vi "get_ROI_boundary.vi"(8 "error in (no error)":errorcluster, 11 "image in":T2) -> (0 "error out":errorcluster, 2 "points":T1[](array[typedef]))   [LabVIEW 2010]
uses:
  <vilib>/vision/Image Controls.llb/IMAQ Image.ctl
  point_cluster.ctl
  <vilib>/vision/NI_Vision_Development_Module.lvlib
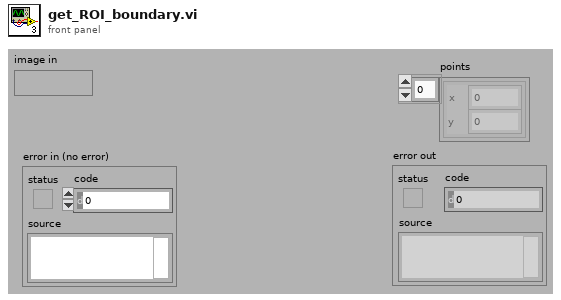
[diagram p1: front panel]
types:
  T1 = typedef "point_cluster.ctl" = cluster{"x":i32, "y":i32}
  T2 = typedef "IMAQ Image.ctl" = refnum<image>
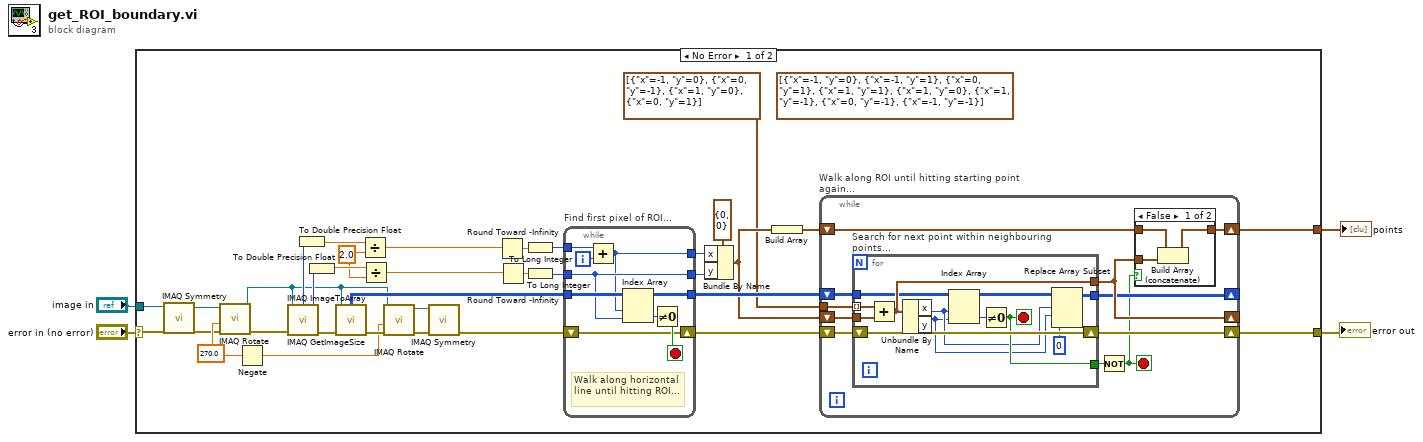
[diagram p0: block diagram]
diagram:
  n1 = case shown="No Error" "error in (no error)" {
    selector: "error in (no error)" -> [w15 w74]
    tunnel: [w26 w74] -> w3
    tunnel: "image in" -> [w13 _]
    tunnel: [w8 _] -> w1
    frame No Error {
      w17 = sgl 270.0 ("Angle (degrees)")
      (unwired) T1[] [{"x"=-1, "y"=0}, {"x"=-1, "y"=1}, {"x"=0, "y"=1}, {"x"=1, "y"=1}, {"x"=1, "y"=0}, {"x"=1, "y"=-1}, {"x"=0, "y"=-1}, {"x"=-1, "y"=-1}]
      w32 = 2.0 ("y")
      n2 = call "IMAQ Symmetry"("error in (no error)"=w15, "Image Src"=w13) -> ("error out"=w14:errorcluster, "Image Dst Out"=w12:T2)  [unwired: 3 in]
      n3 = call "IMAQ Rotate"("error in (no error)"=w14, "Angle (degrees)"=w17, "Image Src"=w12) -> ("error out"=w20:errorcluster, "Image Dst Out"=w18:T2)  [unwired: 7 in]
      n4 = Negate(x=w17) -> (-x=w16:sgl)
      n5 = call "IMAQ GetImageSize"("Image"=w18, "error in (no error)"=w20) -> ("Y Resolution"=w37:i32, "X Resolution"=w38:i32, "error out"=w39:errorcluster)  [unwired: 2 in]
      n6 = To Double Precision Float(number=w38) -> (double precision float=w36:dbl)
      n7 = To Double Precision Float(number=w37) -> (double precision float=w35:dbl)
      n8 = call "IMAQ ImageToArray"("error in (no error)"=w39, "Image"=w18) -> ("error out"=w19:errorcluster, "Image Pixels (U8)"=w22:u8[][])  [unwired: 2 in, 3 out]
      n9 = Divide(x=w36, y=w32) -> (x/y=w34:dbl)
      n10 = Divide(x=w35, y=w32) -> (x/y=w33:dbl)
      n11 = call "IMAQ Rotate"("error in (no error)"=w19, "Angle (degrees)"=w16, "Image Src"=w18) -> ("error out"=w11:errorcluster, "Image Dst Out"=w9:T2)  [unwired: 7 in]
      n12 = call "IMAQ Symmetry"("error in (no error)"=w11, "Image Src"=w9) -> ("error out"=w10:errorcluster)  [unwired: 3 in, 1 out]
      n13 = Round Toward -Infinity(1:w34) -> (0:w31:dbl)
      n14 = Round Toward -Infinity(1:w33) -> (0:w30:dbl)
      n15 = To Long Integer(number=w31) -> (32bit integer=w24:i32)
      n16 = To Long Integer(number=w30) -> (32bit integer=w23:i32)
      n17 = while "Find first pixel of ROI..." {
        tunnel: w22 -> [w68]
        tunnel: w24 -> [w73]
        tunnel: w23 -> [w67]
        shift-right: [w69] -> w29
        shift-left: w10 -> [w69]
        tunnel: [w67] -> w27
        tunnel: [w66] -> w21
        tunnel: [w68] -> w25
        i -> [w72]
        stop <- w70 stop-if-true
        # "Walk along horizontal line until hitting ROI..."
        n18 = Add(x=w73, y=w72) -> (x+y=w66:i32)
        n19 = Index Array(array=w68, index (row)=w66, index (col)=w67) -> (element=w71:u8)
        n20 = Not Equal To 0?(x=w71) -> (x != 0?=w70:bool)
      }
      n21 = Bundle By Name(cluster=T1 {"x"=0, "y"=0} ("point"), "x"=w21, "y"=w27) -> (w6:T1)
      n22 = Build Array(w6) -> (w7:T1[])
      n23 = while "Walk along ROI until hitting starting point again..." {
        shift-right: [w44] -> w8
        shift-left: w7 -> [w45]
        shift-right: [w49] -> w26
        shift-left: w29 -> [w50]
        tunnel: T1[] [{"x"=-1, "y"=0}, {"x"=0, "y"=-1}, {"x"=1, "y"=0}, {"x"=0, "y"=1}] -> [w48]
        shift-right: [w43] -> _
        shift-left: w6 -> [w47]
        shift-right: [w41] -> _
        shift-left: w25 -> [w46]
        stop <- w40 stop-if-true
        n24 = for "Search for next point within neighbouring points..." {
          shift-right: [w62] -> w49
          shift-left: w50 -> [w62]
          tunnel: w48 -> [w65] mode=indexing
          tunnel: w47 -> [w64]
          tunnel: w46 -> [w59]
          tunnel: [w63] -> w43
          tunnel: [w61] -> w42
          tunnel: [w58] -> w41
          stop <- w61 stop-if-true
          n25 = Add(x=w65, y=w64) -> (x+y=w63:T1)
          n26 = Unbundle By Name(w63) -> ("x"=w56:i32, "y"=w55:i32)
          n27 = Index Array(array=w59, index (row)=w56, index (col)=w55) -> (element=w60:u8)
          n28 = Not Equal To 0?(x=w60) -> (x != 0?=w61:bool)
          n29 = Replace Array Subset(array=w59, new element=u8 0, index (row)=w56, index (col)=w55) -> (w58:u8[][])
        }
        n30 = Not(x=w42) -> (.not. x?=w40:bool)
        n31 = case shown="False" w40 {
          tunnel: w45 -> [w53 w54]
          tunnel: [w52 w54] -> w44
          tunnel: w43 -> [w51 _]
          frame False {
            n32 = Build Array (concatenate)(w53, w51) -> (w52:T1[])
          }
          frame True {
          }
        }
      }
    }
    frame Error {
    }
  }
  "points" <- w1
  "error out" <- w3
